vi "POLL BIAS.vi"(8 "error in (no error)":errorcluster, 9 "element":T1 {"Avoid zero threshold (V)" format="%#_13g"}, 10 "ScanQ in":refnum<queue>, 11 "SweepQ in":refnum<queue>) -> (0 "error out":errorcluster, 2 "ScanQ out":refnum<queue>, 3 "SweepQ Out":refnum<queue>)   [LabVIEW 2025]
uses:
  <userlib>/Nanonis Prog Interface V5e/Nanonis Prog Interface.lvlib
  Labview-File/QMH (STM Auto)/CTL's/Scan_Params (QMH).ctl
  Downloads/Magnet Array.ctl
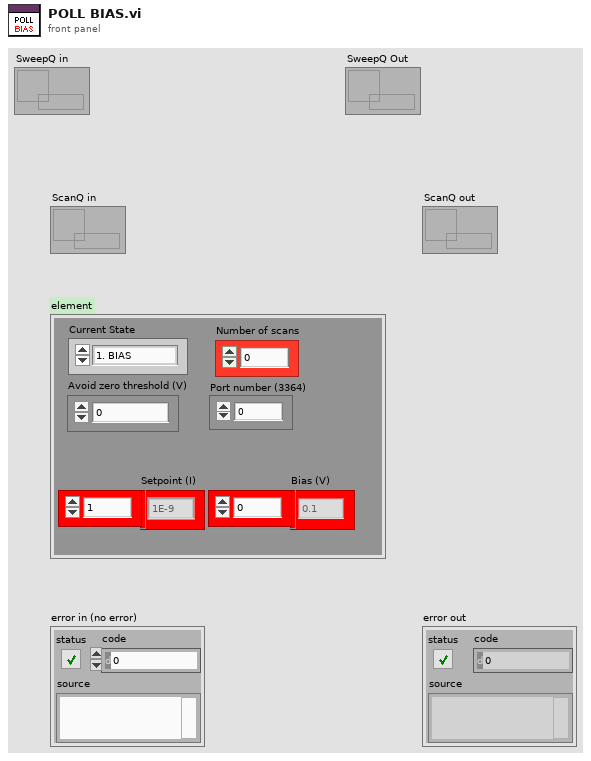
[diagram p1: front panel]
types:
  T1 = typedef "Scan_Params (QMH).ctl" = cluster{"Setpoint (I)":dbl[], "Bias (V)":dbl[], "Number of scans":u8, "Port number (3364)":u32, "Avoid zero threshold (V)":dbl, "Current State":enum16{"1. BIAS", "2. INIT_SCAN", "3. SCAN_IDLE", "4. INTER_SCAN", "5. NEW_COORDS_&_FRAME", "6. FINAL_SCAN", "7. POLL BIAS", "8. Z-CONT", "9. STOP"}}
  T2 = enum16{"1. BIAS", "2. INIT_SCAN", "3. SCAN_IDLE", "4. INTER_SCAN", "5. NEW_COORDS_&_FRAME", "6. FINAL_SCAN", "7. POLL_BIAS", "8. Z-CONT.", "9. STOP"}
  T3 = enum16{"SET FIELD", "SWEEP IDLE", "NEXT FIELD", "SWEEP DONE"}
  T4 = typedef "Magnet Array.ctl" = cluster{"Sweep States":enum16{"SET FIELD", "SWEEP IDLE", "NEXT FIELD", "SWEEP DONE"}, "VISA Connection":refnum<visa-resource-name>, "Fields(T)":dbl[]}
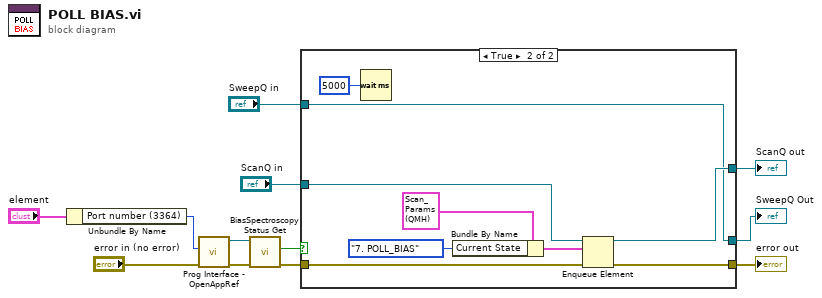
[diagram p0: block diagram]
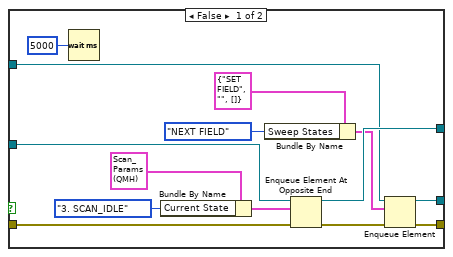
[diagram p2: hidden frame]
diagram:
  n1 = Unbundle By Name("element") -> ("Port number (3364)"=w3:u32)
  n2 = call <userlib>:"Prog Interface - OpenAppRef.vi"("Error in (no error)"="error in (no error)", "Port number (3364)"=w3) -> ("Error out"=w6:errorcluster, "Application reference"=w5:refnum<vi>)  [unwired: 4 in]
  n3 = call <userlib>:"BiasSpectroscopy Status Get.vi"("Error in (no error)"=w6, "Application ref in"=w5) -> ("Error out"=w11:errorcluster, "Running?"=w7:bool)  [unwired: 5 in, 1 out]
  n4 = case shown="True" w7 {
    tunnel: "ScanQ in" -> [w26 w35]
    tunnel: [w23 w32] -> w9
    tunnel: [w22 w29] -> w2
    tunnel: [w20 w30] -> w10
    tunnel: w11 -> [w19 w31]
    tunnel: "SweepQ in" -> [w18 w29]
    frame False {
      n5 = Wait (ms)(milliseconds to wait=u32 5000) -> ()  [unwired: 1 out]
      n6 = Bundle By Name(cluster=T1 {"Setpoint (I)"=[], "Bias (V)"=[], "Number of scans"=1, "Port number (3364)"=3364, "Avoid zero threshold (V)"=0.004999999888241291, "Current State"=enum."1. BIAS"} ("element"), "Current State"=T2."3. SCAN_IDLE") -> (w24:T1)
      n7 = Bundle By Name(cluster=T4 {"Sweep States"=enum."SET FIELD", "VISA Connection"="", "Fields(T)"=[]} ("element"), "Sweep States"=T3."NEXT FIELD") -> (w15:T4)
      n8 = Enqueue Element At Opposite End(queue=w26, element=w24, error in (no error)=w19) -> (queue out=w23:refnum<queue>, error out=w21:errorcluster)  [unwired: 1 in, 1 out]
      n9 = Enqueue Element(queue=w18, element=w15, error in (no error)=w21) -> (queue out=w22:refnum<queue>, error out=w20:errorcluster)  [unwired: 1 in, 1 out]
    }
    frame True {
      n10 = Wait (ms)(milliseconds to wait=u32 5000) -> ()  [unwired: 1 out]
      n11 = Bundle By Name(cluster=T1 {"Setpoint (I)"=[], "Bias (V)"=[], "Number of scans"=1, "Port number (3364)"=3364, "Avoid zero threshold (V)"=0.004999999888241291, "Current State"=enum."1. BIAS"} ("element"), "Current State"=T2."7. POLL_BIAS") -> (w33:T1)
      n12 = Enqueue Element(queue=w35, element=w33, error in (no error)=w31) -> (queue out=w32:refnum<queue>, error out=w30:errorcluster)  [unwired: 1 in, 1 out]
    }
  }
  "error out" <- w10
  "ScanQ out" <- w9
  "SweepQ Out" <- w2
